vi "S8300E_CPU_Threading_WIH.vi"() -> ()   [LabVIEW 2011]
panel:
  out "temp-log2":string
  out "log2":string
  out "LOG1":string
  out "FinalLOG1":string
  out "CMDList":cluster{string, string, string}[](array[cluster])
  out "log msg":string
  out "VISA resource name out":refnum<visa-resource-name>
  out "BEGIN TIME":u32
  out "進行狀況":string
  # "2015-6-1"
  # "S8300E Check CPU Thread(接UART COM9)"
  # "Error Code:CPU-THREAD"
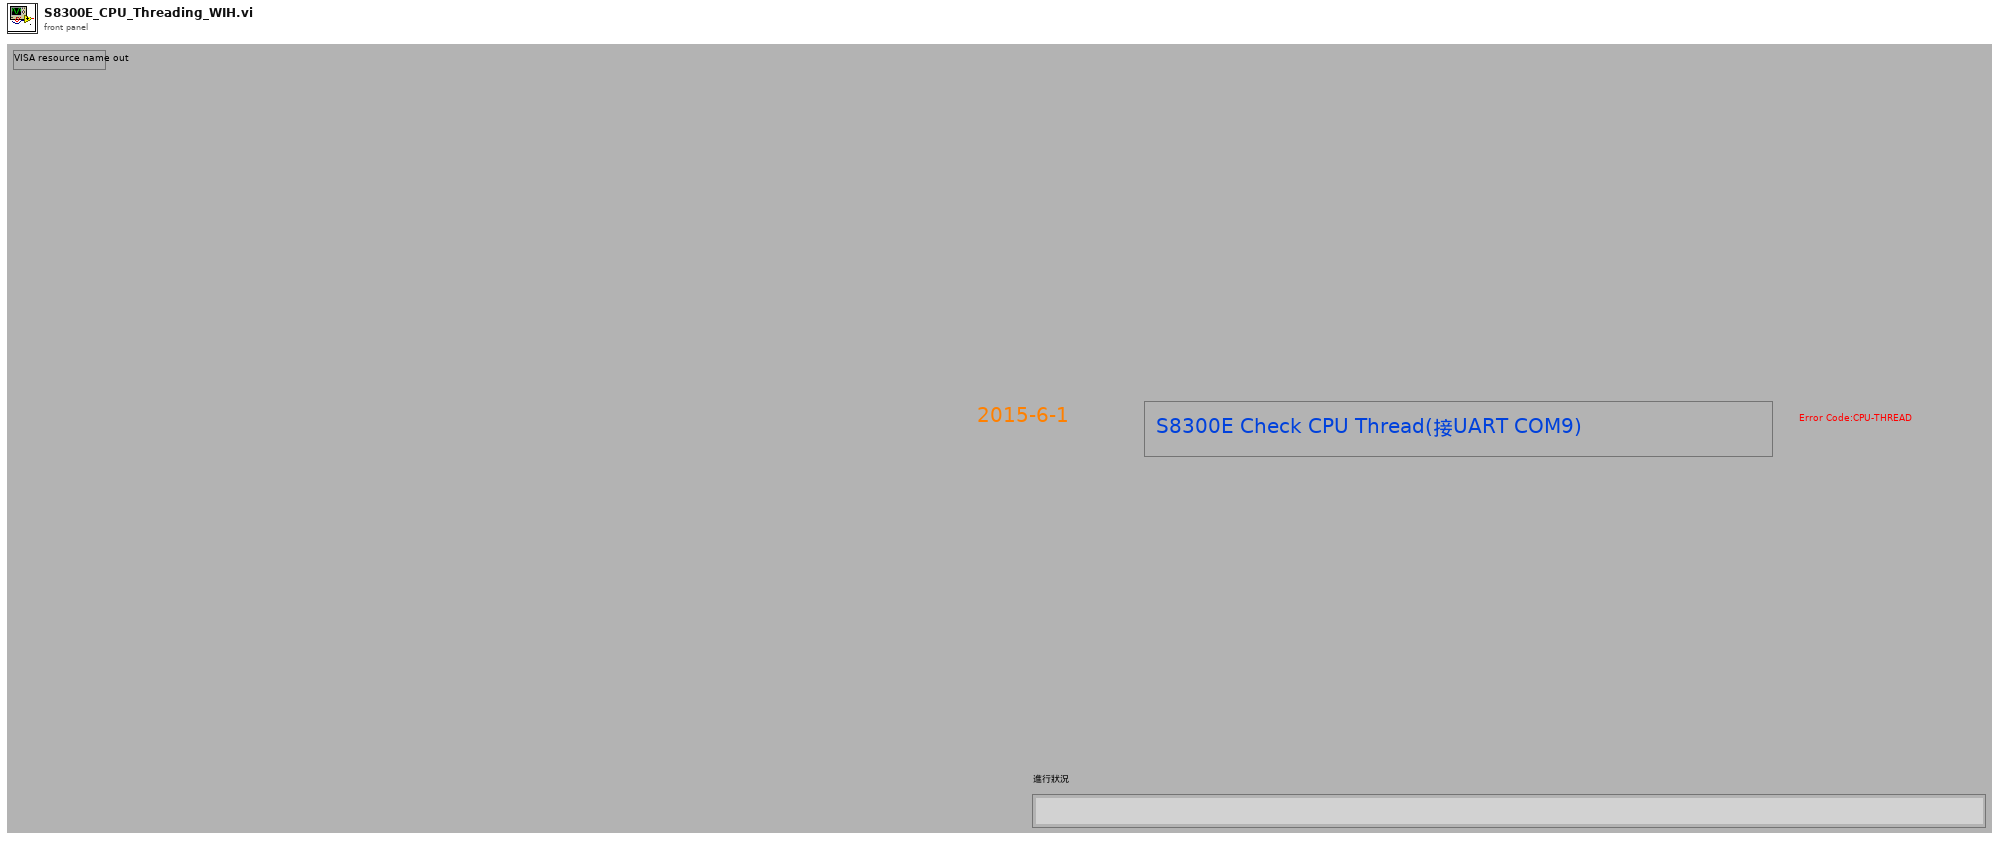
[diagram p1: front panel]
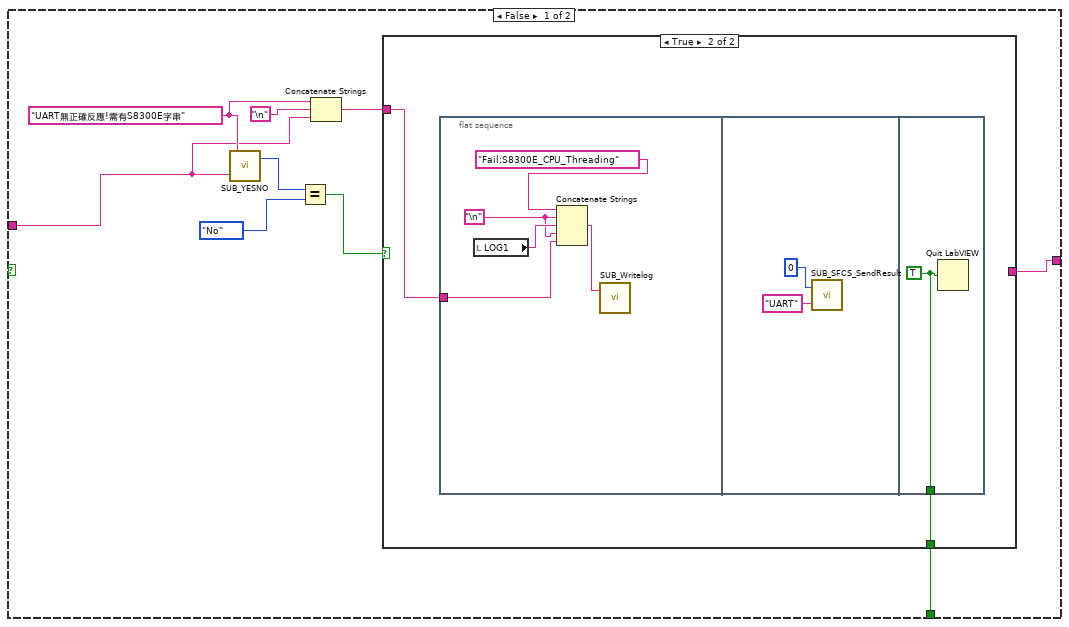
[diagram p4: hidden frame]
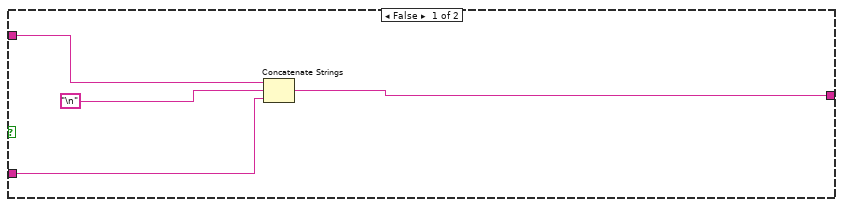
[diagram p6: hidden frame]
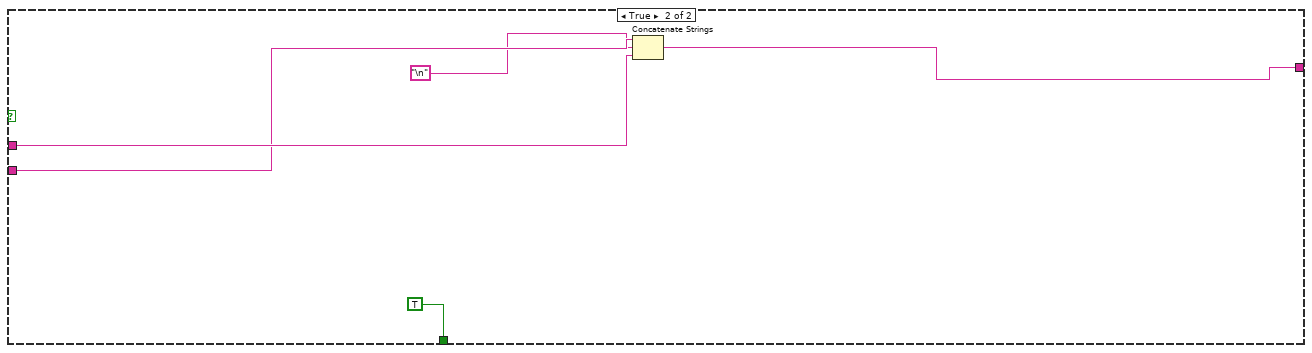
[diagram p7: hidden frame]
diagram:
  n1 = flat-sequence {
    frame #0 {
      n2 = Tick Count (ms)() -> (millisecond timer value=→"BEGIN TIME":u32)
    }
    frame #1 {
      n3 = property on="進行狀況" class="Str"("Blinking"=TRUE) -> ()  [unwired: 2 in, 2 out]
      "進行狀況" <- "進入測試準備中...." ("進行狀況")
    }
    frame #2 {
      n4 = call "SUB_SearchFile_inFolder.vi"("Search Filename in Folder"="S8300E_sfcs_misc.txt") -> ("File Existing True/Flase"=w4:bool)  [unwired: 1 in]
      n5 = case shown="False" w4 {
        frame False {
          n6 = flat-sequence {
            frame #0 {
              n7 = call "Display Message to User"() -> ()  [unwired: 10 in, 2 out]
            }
            frame #1 {
              n8 = call "SUB_Writelog.vi"("Pass/Fail"="Fail:S8300E_CPU_Threading") -> ()  [unwired: 2 in]
            }
            frame #2 {
              n9 = Quit LabVIEW(quit? (T)=TRUE) -> ()
            }
          }
        }
        frame True {
        }
      }
    }
    frame #3 {
      n10 = Concatenate Strings("./cpu.sh -t", "\r") -> (w12:string)
      n11 = Bundle(w12, "PASSED=4", "Checking CPU Threading  Number") -> (w10:cluster{string, string, string})  [unwired: 1 in]
      n12 = Build Array(w10) -> (→"CMDList":cluster{string, string, string}[])
    }
    frame #4 {
      n13 = call "SUB_COM1_CLOSE.vi"("VISA resource name"=refnum<visa-resource-name> "COM9") -> ()  [unwired: 3 in]
    }
    frame #5 {
      n14 = case shown="True" TRUE {
        frame False {
        }
        frame True {
          n15 = call "SUB_COM9_INIT.vi"("baud rate"=u32 115200) -> ("VISA resource name out"=w20:refnum<visa-resource-name>)  [unwired: 1 in, 1 out]
          "VISA resource name out" <- w20
          n16 = call "SUB_COM1Wrt.vi"("VISA resource name"=w20, "write buffer"="\r") -> ("duplicate VISA resource name"=w17:refnum<visa-resource-name>)  [unwired: 1 in, 1 out]
          n17 = call "SUB_ContinueCom1Read.vi"("Numeric"=1200, "duplicate VISA resource name 2"=w17) -> ()  [unwired: 1 in, 3 out]
        }
      }
    }
    frame #6 {
      n18 = while {
        shift-right: [w26] -> w22
        shift-left: "" -> [w25]
        stop <- w36 stop-if-true
        n19 = local read "VISA resource name out"() -> (w28:refnum<visa-resource-name>)
        n20 = call "SUB_ContinueCom1Read.vi"("Numeric"=1200, "duplicate VISA resource name 2"=w28) -> ("duplicate VISA resource name"=w27:refnum<visa-resource-name>)  [unwired: 1 in, 2 out]
        n21 = call "SUB_COM1Wrt.vi"("VISA resource name"=w27, "write buffer"="\r") -> ("duplicate VISA resource name"=w35:refnum<visa-resource-name>)  [unwired: 1 in, 1 out]
        n22 = Tick Count (ms)() -> (millisecond timer value=w34:u32)
        n23 = call "SUB_READ_COM1_FindString_timeout.vi"("Find this String"="s8300e_func_test#", "Timeout Seccond"=3.0, "Begin time"=w34, "duplicate VISA resource name 2"=w35) -> ("Output String"=w30:string, "Found String"=w31:bool)  [unwired: 1 in, 1 out]
        n24 = case shown="True" w31 {
          tunnel: [w43 TRUE] -> w36
          tunnel: w30 -> [w40 w60]
          tunnel: [w38 w58] -> w24
          frame False {
            w42 = "UART無正確反應!需有S8300E字串" ("Status")
            n25 = call "SUB_YESNO.vi"("Debug View"=w40, "Status"=w42) -> ("yes/no"=w46:enum32{"No Selection", "Yes", "No", "None"})  [unwired: 1 in]
            n26 = Equal?(x=w46, y=enum32{"No Selection", "Yes", "No", "None"}."No") -> (x = y?=w44:bool)
            n27 = Concatenate Strings(w42, "\n", w40) -> (w39:string)
            n28 = case shown="True" w44 {
              tunnel: [_ w49] -> w43
              tunnel: w39 -> [w47 w48]
              tunnel: [w47 _] -> w38
              frame False {
              }
              frame True {
                n29 = flat-sequence {
                  tunnel: w48 -> [w51]
                  tunnel: [w57] -> w49
                  frame #0 {
                    w52 = "\n"
                    n30 = local read "LOG1"() -> (w53:string)
                    n31 = Concatenate Strings("Fail:S8300E_CPU_Threading" ("Pass/Fail"), w52, w53, w52, w51) -> (w50:string)
                    n32 = call "SUB_Writelog.vi"("Pass/Fail"=w50) -> ()  [unwired: 2 in]
                  }
                  frame #1 {
                    n33 = call "SUB_SFCS_SendResult.vi"("ErrorCode"="UART", "PASS_Fail (1/0)"=i8 0) -> ()  [unwired: 1 out]
                  }
                  frame #2 {
                    w57 = TRUE ("quit? (T)")
                    n34 = Quit LabVIEW(quit? (T)=w57) -> ()
                  }
                }
              }
            }
          }
          frame True {
            n35 = Concatenate Strings(w60, "\n") -> (w58:string)
          }
        }
        n36 = Concatenate Strings(w25, w24) -> (w26:string)
        "LOG1" <- w26
      }
      "FinalLOG1" <- w22
    }
    frame #7 {
      n37 = local write "log msg"("") -> ()
    }
    frame #8 {
      n38 = local read "CMDList"() -> (w63:cluster{string, string, string}[])
      n39 = Array Size(array=w63) -> (size(s)=w66:i32)
      n40 = for {
        N: w66 -> [_]
        shift-right: [w69] -> w64
        shift-left: "" -> [w67]
        i -> [w71]
        n41 = while {
          tunnel: w71 -> [w87]
          shift-right: [w75] -> w68
          shift-left: "" -> [w74]
          stop <- w81 stop-if-true
          n42 = local read "VISA resource name out"() -> (w83:refnum<visa-resource-name>)
          n43 = local read "CMDList"() -> (w78:cluster{string, string, string}[])
          n44 = Index Array(array=w78, index=w87) -> (element=w79:cluster{string, string, string})
          n45 = Unbundle(w79) -> (w72:string, w76:string, w77:string)
          n46 = call "SUB_COM1Wrt.vi"("VISA resource name"=w83, "write buffer"=w72) -> ("duplicate VISA resource name"=w86:refnum<visa-resource-name>)  [unwired: 1 in, 1 out]
          n47 = Tick Count (ms)() -> (millisecond timer value=w85:u32)
          n48 = call "SUB_READ_COM1_FindString_timeout.vi"("Find this String"=w76, "Timeout Seccond"=3.0, "Begin time"=w85, "duplicate VISA resource name 2"=w86) -> ("Output String"=w80:string, "Found String"=w82:bool)  [unwired: 1 in, 1 out]
          n49 = local write "進行狀況"(w77) -> ()
          n50 = case shown="False" w82 {
            tunnel: [_ TRUE] -> w81
            tunnel: w80 -> [w89 w115]
            tunnel: [w88 w114] -> w73
            tunnel: w72 -> [_ w113]
            frame False {
              w90 = "測試失敗!CPU Thread 須4" ("string")
              n51 = call "SUB_YESNO.vi"("Debug View"=w89, "Status"=w90) -> ("yes/no"=w93:enum32{"No Selection", "Yes", "No", "None"})  [unwired: 1 in]
              n52 = Equal?(x=w93, y=enum32{"No Selection", "Yes", "No", "None"}."No") -> (x = y?=w91:bool)
              n53 = case shown="True" w91 {
                tunnel: w90 -> [w97 w99]
                tunnel: w89 -> [w95 w98]
                tunnel: [w94 _] -> w88
                frame False {
                  n54 = Concatenate Strings(w97, "\n", w95) -> (w94:string)
                }
                frame True {
                  n55 = flat-sequence {
                    tunnel: w99 -> [w106]
                    tunnel: w98 -> [w105]
                    frame #0 {
                      w100 = "\n"
                      w102 = "\n"
                      n56 = local read "temp-log2"() -> (w104:string)
                      n57 = local read "log2"() -> (w103:string)
                      n58 = Concatenate Strings(w106, w100, w105, w100) -> (w101:string)
                      n59 = Concatenate Strings("Fail:S8300E_CPU_Threading" ("Pass/Fail"), w102, w104, w102, w103, w102, w101) -> (w107:string)
                      n60 = call "SUB_Writelog.vi"("Pass/Fail"=w107) -> ()  [unwired: 2 in]
                    }
                    frame #1 {
                      n61 = call "SUB_SFCS_SendResult.vi"("ErrorCode"="CPU-THREAD", "PASS_Fail (1/0)"=i8 0) -> ()  [unwired: 1 out]
                    }
                    frame #2 {
                      n62 = Quit LabVIEW(quit? (T)=TRUE) -> ()
                    }
                  }
                }
              }
            }
            frame True {
              n63 = Concatenate Strings(w113, "\n", w115) -> (w114:string)
            }
          }
          n64 = Concatenate Strings(w74, w73) -> (w75:string)
          "log2" <- w75
        }
        n65 = Concatenate Strings(w67, w68) -> (w69:string)
        "temp-log2" <- w69
      }
      "log msg" <- w64
    }
    frame #9 {
      n66 = call "SUB_COM1_CLOSE.vi"("VISA resource name"=refnum<visa-resource-name> "COM9") -> ()  [unwired: 3 in]
    }
    frame #10 {
      w120 = "***Not Good ***" ("replace string (\"\")")
      w125 = "\n"
      n67 = local read "FinalLOG1"() -> (w127:string)
      n68 = local read "log msg"() -> (w126:string)
      n69 = local read "BEGIN TIME"() -> (w130:u32)
      n70 = Tick Count (ms)() -> (millisecond timer value=w129:u32)
      n71 = call "SUB_CAL_TESTTIME.vi"("Test Item name"="S8300E_CPU_Threading", "Stop tick time"=w129, "Start tick time"=w130) -> ("Test Time output"=w124:string)  [unwired: 2 in]
      n72 = Concatenate Strings("Pass:S8300E_CPU_Threading", w125, w127, w125, w126, w125, w124) -> (w119:string)
      n73 = call "SUB_SEARCH_REPLACE_STR.vi"("replace string (\"\")"=w120, "search string"="FAILED", "input string"=w119) -> ("result string"=w122:string)  [unwired: 2 in]
      n74 = call "SUB_SEARCH_REPLACE_STR.vi"("replace string (\"\")"=w120, "search string"="FAIL", "input string"=w122) -> ("result string"=w118:string)  [unwired: 2 in]
      n75 = call "SUB_Writelog.vi"("Pass/Fail"=w118) -> ()  [unwired: 2 in]
    }
    frame #11 {
      n76 = Request Deallocation(TRUE ("flag")) -> ()
    }
    frame #12 {
      n77 = Quit LabVIEW(quit? (T)=TRUE ("stop? (T)")) -> ()
    }
  }
